vi "CfgManager Test Launcher.vi"() -> ()   [LabVIEW 2013]
uses:
  source/Cache/ConfigManager.Cache.lvclass
  source/Manager/Decompose KVPs.vi
  source/Manager/ConfigManager.lvclass
panel:
  out "Read/Write Passed":bool
  out "Cluster":errorcluster
  out "keys listed":string[](array[string])
  out "keys written":string[](array[string])
  out "Values":variant[](array[variant])
  out "keys read":string[](array[string])
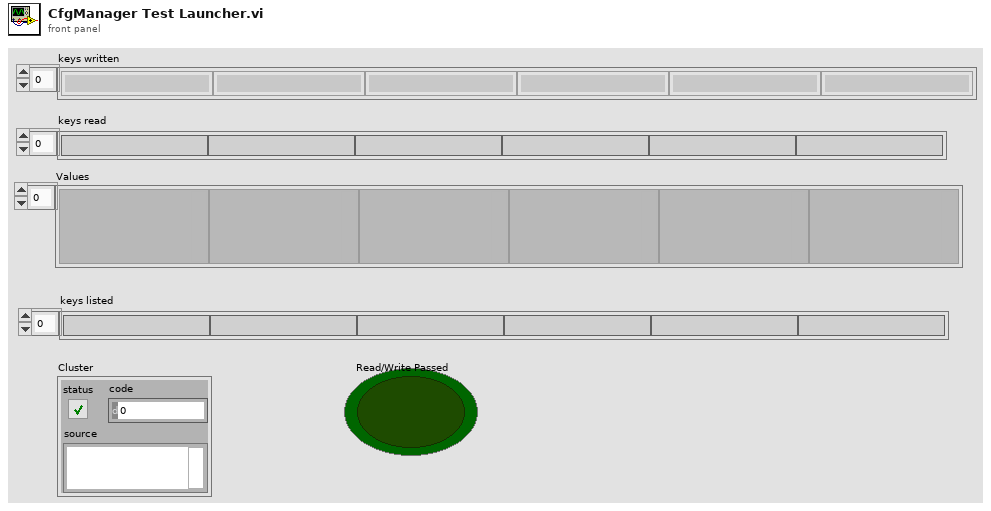
[diagram p1: front panel]
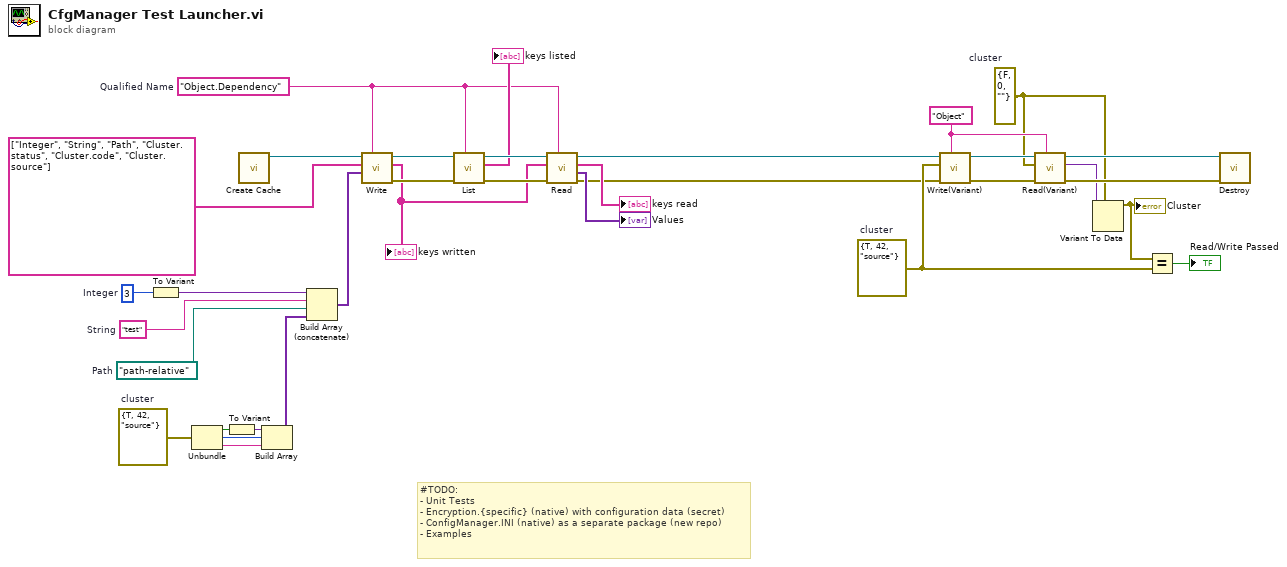
[diagram p0: block diagram]
diagram:
  w5 = errorcluster {"status"=TRUE, "code"=42, "source"="source"}  # cluster
  w4 = errorcluster {"status"=FALSE, "code"=0, "source"=""}  # cluster
  w10 = "Object" ("Name")
  w1 = "Object.Dependency"  # Qualified Name
  w6 = errorcluster {"status"=TRUE, "code"=42, "source"="source"}  # cluster
  w28 = path "path-relative"  # Path
  w29 = "test"  # String
  w31 = 3  # Integer
  # "#TODO: \n- Unit Tests\n- Encryption.{specific} (native) with configuration data (secret)\n- ConfigManager.INI (native) as a separate package (new repo)\n- Examples"
  n1 = To Variant(anything=w31) -> (Variant=w30:variant)
  n2 = Unbundle(w6) -> ("status"=w19:bool, "code"=w18:i32, "source"=w17:string)
  n3 = To Variant(anything=w19) -> (Variant=w16:variant)
  n4 = call "Create Cache.vi"() -> ("ConfigManager.Cache"=w32:refnum<class "ConfigManager.Cache.lvclass">)  [unwired: 11 in]
  n5 = Build Array(w16, w18, w17) -> (w15:variant[])
  n6 = Build Array (concatenate)(w30, w29, w28, w15) -> (w27:variant[])
  n7 = call "Write.vi"("Qualified Name"=w1, "Values"=w27, "keys"=string[] ["Integer", "String", "Path", "Cluster.status", "Cluster.code", "Cluster.source"] ("keys written"), "ConfigManager in"=w32) -> ("error out"=w24:errorcluster, "keys dup"=w20:string[], "ConfigManager out"=w26:refnum<class "ConfigManager.Cache.lvclass">)  [unwired: 5 in]
  "keys written" <- w20
  n8 = call "List.vi"("Qualified Name"=w1, "error in (no error)"=w24, "ConfigManager in"=w26) -> ("error out"=w23:errorcluster, "Keys"=→"keys listed":string[], "ConfigManager out"=w25:refnum<class "ConfigManager.Cache.lvclass">)  [unwired: 6 in]
  n9 = call "Read.vi"("Qualified Name"=w1, "error in (no error)"=w23, "keys in"=w20, "ConfigManager in"=w25) -> ("error out"=w3:errorcluster, "Values"=→"Values":variant[], "keys"=→"keys read":string[], "ConfigManager out"=w2:refnum<class "ConfigManager.Cache.lvclass">)  [unwired: 2 in, 2 out]
  n10 = call "Write(Variant).vi"("Qualified Name"=w10, "error in (no error)"=w3, "value"=w5, "ConfigManager in"=w2) -> ("error out"=w12:errorcluster, "ConfigManager out"=w14:refnum<class "ConfigManager.Cache.lvclass">)  [unwired: 5 in, 1 out]
  n11 = call "Read(Variant).vi"("Qualified Name"=w10, "error in (no error)"=w12, "Type"=w4, "ConfigManager in"=w14) -> ("error out"=w11:errorcluster, "value"=w9:variant, "ConfigManager out"=w13:refnum<class "ConfigManager.Cache.lvclass">)  [unwired: 3 in, 2 out]
  n12 = Variant To Data(type=w4, Variant=w9) -> (data=w8:errorcluster)  [unwired: 1 in, 1 out]
  "Cluster" <- w8
  n13 = Equal?(x=w8, y=w5) -> (x = y?=→"Read/Write Passed":bool)
  n14 = call-dynamic "Destroy.vi"("error in (no error)"=w11, "ConfigManager.Cache in"=w13) -> ()  [unwired: 8 in, 2 out]
